vi "Acknowledging Dialog.vi"(8 "error in (no error)":errorcluster, 9 "Comment":string, 10 "User":string="(Nobody)") -> (0 "error out":errorcluster, 1 "Comment Out":string, 2 "User Out":string, 3 "Cancelled?":bool)   [LabVIEW 2024]
doc: "This VI is a user interface VI and is used to get the acknowledging information."
panel:
  in  "Cancel":bool
  in  "OK":bool
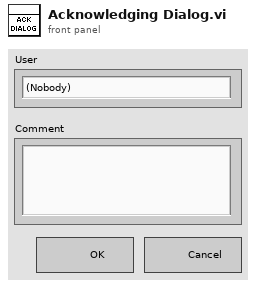
[diagram p1: front panel]
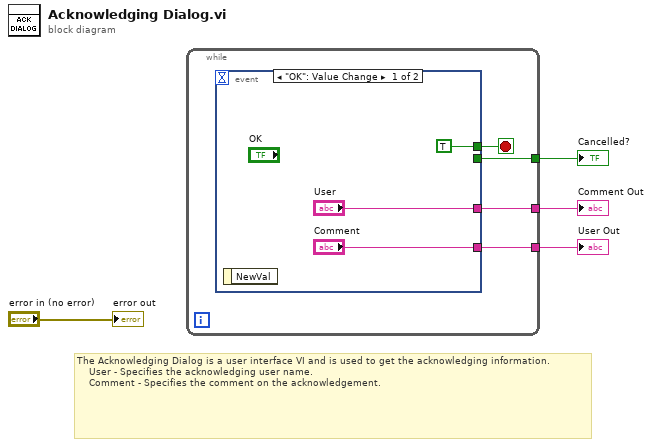
[diagram p0: block diagram]
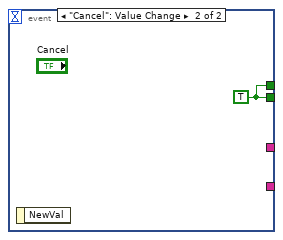
[diagram p2: hidden frame]
diagram:
  # "The Acknowledging Dialog is a user interface VI and is used to get the acknowledging information.\n    User - Specifies the acknowledging user name. \n    Comment - Specifies the comment on the acknowledgement."
  n1 = while {
    tunnel: [w7] -> w3
    tunnel: [w6] -> w2
    tunnel: [w5] -> w1
    stop <- w8 stop-if-true
    n2 = event shown="[0] \"OK\": Value Change" {
      selector: _ -> [_ _]
      dyn-events: _ -> [_ _]
      timeout: _ -> [_ _]
      tunnel: [TRUE w12] -> w8
      tunnel: [_ w12] -> w5
      tunnel: ["Comment" _] -> w6
      tunnel: ["User" _] -> w7
      event "OK": Value Change {
        n3 = event-data() -> ()  [unwired: 1 in, 1 out]
      }
      event "Cancel": Value Change {
        w12 = TRUE
        n4 = event-data() -> ()  [unwired: 1 in, 1 out]
      }
    }
  }
  "User Out" <- w2
  "Comment Out" <- w3
  "Cancelled?" <- w1
  "error out" <- "error in (no error)"
